vi "Write Value.vi"(8 "error in (no error)":errorcluster, 10 "Data":T1, 11 "Numeric in":refnum<class "Const_U8_1D.lvclass">) -> (0 "error out":errorcluster, 3 "Numeric out":refnum<class "Const_U8_1D.lvclass">)   [LabVIEW 2021, in "Const_U8_1D.lvclass"]
uses:
  Const_U8_1D.lvclass
  Type.ctl
  Const_U8_1D.lvclass/Const_U8_1D.ctl
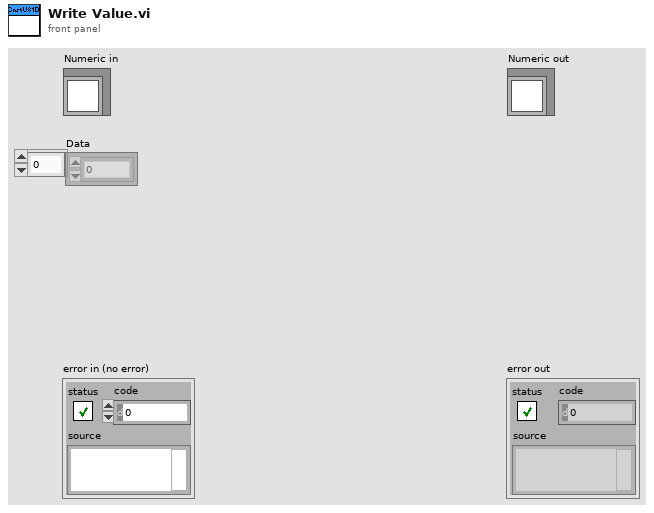
[diagram p1: front panel]
types:
  T1 = typedef "Const_U8_1D.lvclass/Type.ctl" = u8[]
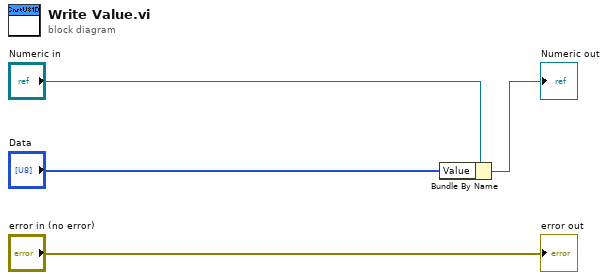
[diagram p0: block diagram]
diagram:
  n1 = Bundle By Name(cluster="Numeric in", "Value"="Data") -> (→"Numeric out":refnum<class "Const_U8_1D.lvclass">)
  "error out" <- "error in (no error)"
